vi "Scan1762ARPPumpingHWT.vi"() -> ()   [LabVIEW 2012]
uses:
  <vilib>/Utility/file.llb/Write To Spreadsheet File (DBL).vi
panel:
  in  "1762 Sweep Width":dbl=100000.0
  out "digital waveform out 3":digitalwaveform(waveform)={"t0"=timestamp(0 s since 1904-01-01), "dt"=1e-07, "Y"={"transitions"=[0, 20000, 21001, 21501, 22501, 42500], "data"=[[1, 1, 0, 0], [0, 0, 0, 0], [0, 0, 0, 1], [0, 0, 0, 0], [1, 1, 0, 0], [1, 1, 0, 0]]}, "error"={"status"=FALSE, "code"=37421928, "source"=""}}
  out "10xwindow":i32
  out "10xdiscr":dbl
  out "DARK?":i32(graph)
  out "Counts":i32
  out "DARK?":bool
  out "PMT Counts":i32(graph)
  in  "PMT sample time":dbl=0.05
  out "Counts after 1762":i32=57
  out "OuterLoop":i32=101
  out "InnerLoop":i32=19
  out "Frequency Step Size":dbl=10000.0
  out "Bright Events":dbl
  in  "Discriminator Level\n (Bright/Dark)":i32=20
  out "digital waveform out 2":digitalwaveform(waveform)={"t0"=timestamp(0 s since 1904-01-01), "dt"=1e-07, "Y"={"transitions"=[0, 20000, 21001, 21501, 22501, 42500], "data"=[[1, 1, 0, 0], [0, 0, 0, 0], [0, 0, 0, 1], [0, 0, 0, 0], [1, 1, 0, 0], [1, 1, 0, 0]]}, "error"={"status"=FALSE, "code"=37421928, "source"=""}}
  in  "1762 Sweep Time (milliseconds)":dbl=0.3
  in  "Comment":string="*@* DPAOM = 84MHz, B-current = 2.91Amps, Comp Coil = 3.00 Amps, Axial Voltage = 500 Volts, RF frequency = 18.115, RF power = -8dBm"
  in  "B Field":dbl=2.26
  in  "Power":dbl
  in  "Rerun BG Every\nnth freq point":dbl=20.0
  in  "PMT sample time":dbl=0.05
  out "Counts finding bright ion":dbl=39.0
  in  "BG Cutoff Limit":dbl=38.0
  in  "Runs per data point":dbl=50.0
  in  "Low Freq":dbl(slide)=80000000.0 min=50000000.0 max=120000000.0 step=1000.0 scale=80000000.0..90000000.0 scale format="%#.5f"
  in  "High Freq":dbl(slide)=90000000.0 min=50000000.0 max=120000000.0 step=1000.0 scale=80000000.0..90000000.0 scale format="%#.0f"
  out "Cur Freq":dbl=85984000.0 format="%#_8f"
  out "Path":path=path "c:/data/1762 Scans/2014-05-20_19-16-05_1762scanWithPumping.txt"
  out "Frequency Scan":cluster{dbl, dbl}[](graph)=[{87004000.0, 1.0}, {86994000.0, 1.0}, {86984000.0, 1.0}, {86974000.0, 1.0}, {86964000.0, 1.0}, {86954000.0, 1.0}, {86944000.0, 1.0}, {86934000.0, 1.0}, {86924000.0, 1.0}, {86914000.0, 1.0}, {86904000.0, 1.0}, {86894000.0, 1.0}, {86884000.0, 1.0}, {86874000.0, 1.0}, {86864000.0, 1.0}, {86854000.0, 1.0}, {86844000.0, 1.0}, {86834000.0, 1.0}, {86824000.0, 1.0}, {86814000.0, 1.0}, {86804000.0, 1.0}, {86794000.0, 1.0}, {86784000.0, 1.0}, {86774000.0, 1.0}, {86764000.0, 1.0}, {86754000.0, 1.0}, {86744000.0, 1.0}, {86734000.0, 1.0}, {86724000.0, 1.0}, {86714000.0, 1.0}, {86704000.0, 1.0}, {86694000.0, 1.0}, {86684000.0, 1.0}, {86674000.0, 1.0}, {86664000.0, 1.0}, {86654000.0, 1.0}, {86644000.0, 1.0}, {86634000.0, 1.0}, {86624000.0, 1.0}, {86614000.0, 1.0}, {86604000.0, 1.0}, {86594000.0, 1.0}, {86584000.0, 1.0}, {86574000.0, 1.0}, {86564000.0, 1.0}, {86554000.0, 1.0}, {86544000.0, 1.0}, {86534000.0, 1.0}, {86524000.0, 1.0}, {86514000.0, 1.0}, {86504000.0, 1.0}, {86494000.0, 1.0}, {86484000.0, 1.0}, {86474000.0, 1.0}, {86464000.0, 1.0}, {86454000.0, 1.0}, {86444000.0, 1.0}, {86434000.0, 1.0}, {86424000.0, 1.0}, {86414000.0, 1.0}, {86404000.0, 1.0}, {86394000.0, 1.0}, {86384000.0, 1.0}, {86374000.0, 1.0}, {86364000.0, 1.0}, {86354000.0, 1.0}, {86344000.0, 1.0}, {86334000.0, 1.0}, {86324000.0, 1.0}, {86314000.0, 1.0}, {86304000.0, 1.0}, {86294000.0, 1.0}, {86284000.0, 1.0}, {86274000.0, 1.0}, {86264000.0, 1.0}, {86254000.0, 1.0}, {86244000.0, 1.0}, {86234000.0, 1.0}, {86224000.0, 1.0}, {86214000.0, 1.0}, {86204000.0, 1.0}, {86194000.0, 1.0}, {86184000.0, 1.0}, {86174000.0, 1.0}, {86164000.0, 1.0}, {86154000.0, 1.0}, {86144000.0, 1.0}, {86134000.0, 1.0}, {86124000.0, 1.0}, {86114000.0, 1.0}, {86104000.0, 1.0}, {86094000.0, 1.0}, {86084000.0, 1.0}, {86074000.0, 1.0}, {86064000.0, 1.0}, {86054000.0, 1.0}, {86044000.0, 1.0}, {86034000.0, 1.0}, {86024000.0, 1.0}, {86014000.0, 1.0}, {86004000.0, 1.0}, {85994000.0, 1.0}]
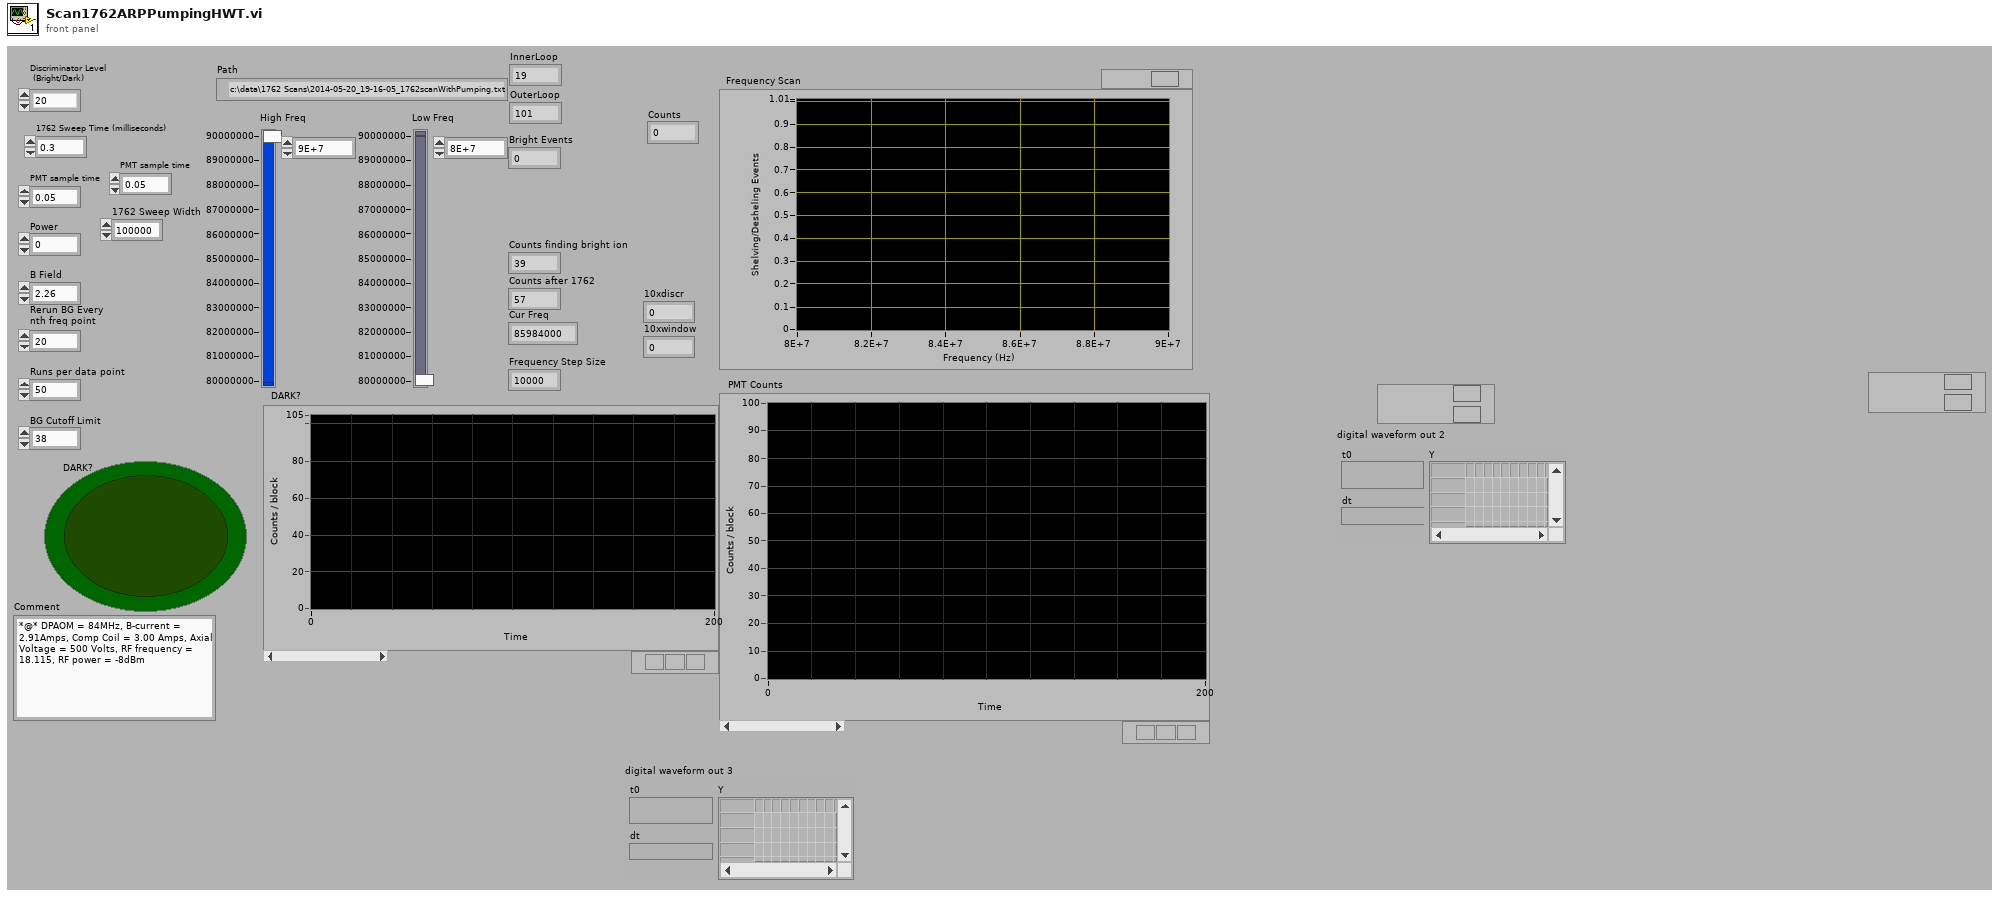
[diagram p1: front panel]
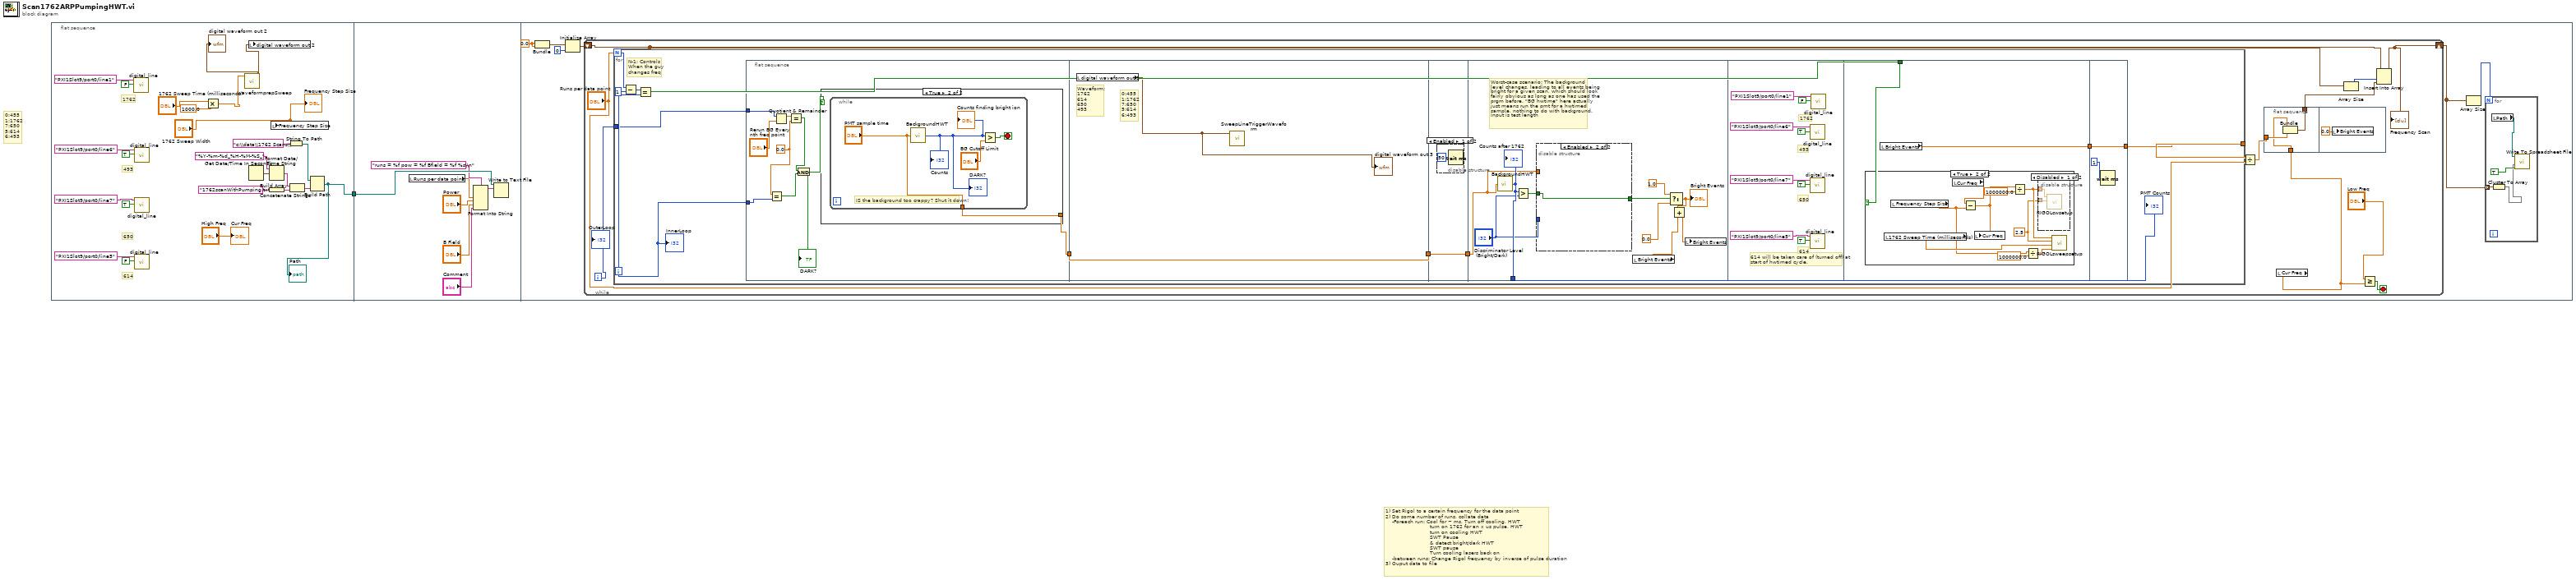
[diagram p0: block diagram]
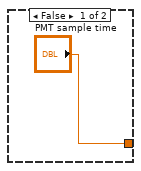
[diagram p2: hidden frame]
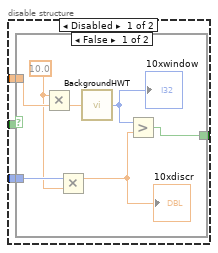
[diagram p4: hidden frame]
diagram:
  # "0:455\n1:1762\n7:650\n5:614\n6:493"
  # "1) Set Rigol to a certain frequency for the data point\n2) Do some number of runs, collate data\n    -Foreach run: Cool for ~ ms, Turn off cooling, HWT\n                           turn on 1762 for an x us pulse, HWT\n                           turn on cooling HWT\n                           SWT Pause\n                           & detect bright/dark HWT\n                           SWT pause\n                           Turn cooling lasers back on \n    -between runs: Change Rigol frequency by inverse of pulse duration\n3) Ouput data to file"
  n1 = flat-sequence {
    tunnel: [w16] -> w1
    tunnel: w1 -> [w31]
    frame #0 {
      # "614"
      # "650"
      # "493"
      # "1762"
      n2 = call "digital_line.vi"("Boolean"=FALSE, "lines"=tag "PXI1Slot9/port0/line1") -> ()  [unwired: 5 in, 1 out]
      n3 = call "digital_line.vi"("Boolean"=TRUE, "lines"=tag "PXI1Slot9/port0/line6") -> ()  [unwired: 5 in, 1 out]
      n4 = call "digital_line.vi"("Boolean"=TRUE, "lines"=tag "PXI1Slot9/port0/line7") -> ()  [unwired: 5 in, 1 out]
      n5 = call "digital_line.vi"("Boolean"=FALSE, "lines"=tag "PXI1Slot9/port0/line5") -> ()  [unwired: 5 in, 1 out]
      n6 = Multiply(x="1762 Sweep Time (milliseconds)", y=1000.0) -> (x*y=w2:dbl)
      n7 = call "waveformprepSweep.vi"("1762 pulse length (units of 1 us)"=w2) -> ("digital waveform out 2"=w6:digitalwaveform)  [unwired: 8 in]
      "digital waveform out 2" <- w6
      n8 = local write "digital waveform out 2"(w6) -> ()
      n9 = Get Date/Time In Seconds() -> (seconds since 1Jan1904=w18:timestamp)
      n10 = Format Date/Time String(time format string (%c)="%Y-%m-%d_%H-%M-%S_", seconds (now)=w18) -> (date/time string=w20:string)  [unwired: 1 in]
      n11 = Build Array("1762scanWithPumping.txt") -> (w23:string[])
      n12 = local write "Frequency Step Size"("1762 Sweep Width") -> ()
      n13 = String To Path(string="c:\\data\\1762 Scans\\") -> (path=w24:path)
      n14 = Concatenate Strings(w20, w23) -> (w22:string)
      n15 = Build Path(base path=w24, name or relative path=w22) -> (appended path=w16:path)
      "Path" <- w16
      "Cur Freq" <- "High Freq"
      "Frequency Step Size" <- "1762 Sweep Width"
    }
    frame #1 {
      n16 = local read "Runs per data point"() -> (w28:dbl)
      n17 = Format Into String(format string="runs = %f pow = %f Bfield = %f %s\\n", w28, "Power", "B Field", "Comment") -> (resulting string=w29:string)  [unwired: 2 in, 1 out]
      n18 = Write to Text File(file (use dialog)=w31, text=w29) -> ()  [unwired: 2 in, 3 out]
    }
    frame #2 {
      w36 = 0.0
      n19 = Bundle(w36, w36) -> (w37:cluster{dbl, dbl})  [unwired: 1 in]
      n20 = Initialize Array(w37, 0) -> (w34:cluster{dbl, dbl}[])
      n21 = while {
        shift-right: [w48] -> w32
        shift-left: w34 -> [w49]
        i -> [w47]
        stop <- w51 stop-if-true
        n22 = for {
          N: "Runs per data point" -> [w65]
          tunnel: [w64] -> w44
          tunnel: w47 -> [w61]
          i -> [w62]
          # "N-1: Controls\nWhen the guy\nchanges freq"
          n23 = Subtract(x=w65, y=1) -> (x-y=w68:i32)
          n24 = Equal?(x=w68, y=w62) -> (x = y?=w66:bool)
          n25 = flat-sequence {
            tunnel: w62 -> [w75]
            tunnel: w61 -> [w70]
            tunnel: [w69] -> w60
            tunnel: [w85] -> w57
            tunnel: w60 -> [w85]
            tunnel: [w86] -> w58
            tunnel: w57 -> [w86]
            tunnel: w58 -> [w90]
            tunnel: [w92] -> w59
            tunnel: w66 -> [w119]
            tunnel: [w120] -> w63
            tunnel: [w133] -> w64
            tunnel: w63 -> [w133]
            frame #0 {
              w74 = 0.0 ("x")
              n26 = Equal?(x=w74, y=w75) -> (x = y?=w72:bool)
              n27 = Quotient & Remainder(x=w70, y="Rerun BG Every\nnth freq point") -> (x-y*floor(x/y)=w76:dbl)  [unwired: 1 out]
              n28 = Equal?(x=w76, y=w74) -> (x = y?=w73:bool)
              n29 = And(x=w73, y=w72) -> (x .and. y?=w71:bool)
              "DARK?" <- w71
              n30 = case shown="True" w71 {
                tunnel: ["PMT sample time" w79] -> w69
                frame False {
                }
                frame True {
                  n31 = while {
                    tunnel: ["PMT sample time"] -> w79
                    stop <- w82 stop-if-true
                    # "IS the background too crappy? Shut it down!"
                    n32 = call "BackgroundHWT.vi"("Sample Time(seconds)"="PMT sample time") -> ("Counts"=w80:i32)
                    "Counts finding bright ion" <- w80
                    "Counts" <- w80
                    "DARK?" <- w80
                    n33 = Greater?(x=w80, y="BG Cutoff Limit") -> (0:w82:bool)
                  }
                }
              }
            }
            frame #1 {
              # "0:455\n1:1762\n7:650\n5:614\n6:493"
              # "Waveform:\n1762\n614\n650\n493"
              n34 = local read "digital waveform out 2"() -> (w84:digitalwaveform)
              "digital waveform out 3" <- w84
              n35 = call "SweepLineTriggerWaveform.vi"("digital waveform in"=w84) -> ()  [unwired: 11 in]
            }
            frame #2 {
              n36 = disable-structure shown="Enabled" {
                frame Enabled {
                  n37 = Wait (ms)(milliseconds to wait=u32 50) -> ()  [unwired: 1 out]
                }
                frame Disabled {
                }
              }
            }
            frame #3 {
              # "Worst-case scenario: The background\nlevel changes, leading to all events being\nbright for a given scan, which should look\nfairly obvious as long as one has used the\nprgm before. \"BG hwtime\" here actually\njust means run the pmt for a hwtimed\nsample, nothing to do with background.\nInput is test length"
              n38 = call "BackgroundHWT.vi"("Sample Time(seconds)"=w90) -> ("Counts"=w92:i32)
              "Counts after 1762" <- w92
              n39 = Greater?(x=w92, y="Discriminator Level\n (Bright/Dark)") -> (0:w91:bool)
              n40 = disable-structure shown="Enabled" {
                disable-tunnel: w91 -> [w101 w110]
                disable-tunnel: [w100 w110] -> w88
                disable-tunnel: w90 -> [w99 _]
                disable-tunnel: "Discriminator Level\n (Bright/Dark)" -> [w98 _]
                frame Disabled {
                  n41 = case shown="False" w101 {
                    selector: w101 -> [_ w109]
                    tunnel: [w104 w109] -> w100
                    tunnel: w99 -> [w108 _]
                    tunnel: w98 -> [w105 _]
                    frame False {
                      w102 = 10.0 ("x")
                      n42 = Multiply(x=w102, y=w108) -> (x*y=w107:dbl)
                      n43 = Multiply(x=w105, y=w102) -> (x*y=w103:dbl)
                      "10xdiscr" <- w103
                      n44 = call "BackgroundHWT.vi"("Sample Time(seconds)"=w107) -> ("Counts"=w106:i32)
                      "10xwindow" <- w106
                      n45 = Greater?(x=w106, y=w103) -> (0:w104:bool)
                    }
                    frame True {
                    }
                  }
                }
                frame Enabled {
                }
              }
              n46 = local read "Bright Events"() -> (w93:dbl)
              n47 = Select(t=1.0, s=w88, f=0.0) -> (s? t:f=w95:dbl)
              "Bright Events" <- w95
              n48 = Add(x=w95, y=w93) -> (x+y=w94:dbl)
              n49 = local write "Bright Events"(w94) -> ()
            }
            frame #4 {
              # "614 will be taken care of (turned off) at\nstart of hwtimed cycle."
              # "614"
              # "650"
              # "493"
              # "1762"
              n50 = call "digital_line.vi"("Boolean"=TRUE, "lines"=tag "PXI1Slot9/port0/line6") -> ()  [unwired: 5 in, 1 out]
              n51 = call "digital_line.vi"("Boolean"=TRUE, "lines"=tag "PXI1Slot9/port0/line7") -> ()  [unwired: 5 in, 1 out]
              n52 = call "digital_line.vi"("Boolean"=TRUE, "lines"=tag "PXI1Slot9/port0/line5") -> ()  [unwired: 5 in, 1 out]
              n53 = call "digital_line.vi"("Boolean"=FALSE, "lines"=tag "PXI1Slot9/port0/line1") -> ()  [unwired: 5 in, 1 out]
            }
            frame #5 {
              n54 = case shown="True" w119 {
                frame False {
                }
                frame True {
                  w125 = 2.5 ("Amplitude (Vpp)")
                  n55 = local read "1762 Sweep Time (milliseconds)"() -> (w124:dbl)
                  n56 = local read "Frequency Step Size"() -> (w123:dbl)
                  n57 = local read "Cur Freq"() -> (w129:dbl)
                  n58 = Subtract(x=w129, y=w123) -> (x-y=w128:dbl)
                  n59 = local write "Cur Freq"(w128) -> ()
                  n60 = Divide(x=w128, y=1000000.0) -> (x/y=w126:dbl)
                  n61 = Divide(x=w123, y=1000000.0) -> (x/y=w122:dbl)
                  n62 = disable-structure shown="Disabled" {
                    disable-tunnel: w125 -> [w131 _]
                    disable-tunnel: w126 -> [w130 _]
                    frame Disabled {
                      n63 = call "RIGOLcwsetup.vi"("Amplitude (Vpp)"=w131, "Frequency (MHz)"=w130) -> ()  [unwired: 10 in]
                    }
                    frame Enabled {
                    }
                  }
                  n64 = call "RIGOLsweepsetup.vi"("AP Sweep Width (MHz)"=w122, "Time (ms)"=w124, "Amplitude (Vpp)"=w125, "Frequency (MHz)"=w126) -> ()  [unwired: 8 in]
                }
              }
              n65 = local read "Bright Events"() -> (w120:dbl)
            }
            frame #6 {
              n66 = Wait (ms)(milliseconds to wait=u32 1) -> ()  [unwired: 1 out]
            }
          }
          "InnerLoop" <- w62
          "PMT Counts" <- w59
        }
        n67 = Divide(x=w44, y="Runs per data point") -> (x/y=w43:dbl)
        n68 = flat-sequence {
          tunnel: w43 -> [w55]
          tunnel: [w54] -> w46
          tunnel: w45 -> [w53]
          frame #0 {
            n69 = Bundle("Cur Freq"=w53, w55) -> (w54:cluster{"Cur Freq":dbl, dbl})  [unwired: 1 in]
          }
          frame #1 {
            n70 = local write "Bright Events"(0.0 ("Bright Events")) -> ()
          }
        }
        n71 = local read "Cur Freq"() -> (w45:dbl)
        n72 = Array Size(array=w49) -> (size(s)=w50:i32)
        n73 = Greater Or Equal?(x="Low Freq", y=w45) -> (x >= y?=w51:bool)
        n74 = Insert Into Array(array=w49, index=w50, new element=w46) -> (w48:cluster{dbl, dbl}[])
        "Frequency Scan" <- w48
        "OuterLoop" <- w47
      }
      n75 = Array Size(array=w32) -> (size(s)=w33:i32)
      n76 = for {
        N: w33 -> [_]
        tunnel: w32 -> [w41] mode=indexing
        n77 = local read "Path"() -> (w38:path)
        n78 = Cluster To Array(cluster=w41) -> (array=w39:dbl[])
        n79 = call-poly <vilib>:"Write To Spreadsheet File.vi"("append to file? (new file:F)"=TRUE, "1D data"=w39, "file path (dialog if empty)"=w38) -> ()  [unwired: 5 in, 1 out]
      }
    }
  }
